vi "Prepend String Length.vi"(7 "String":string, 9 "byte order":T1(ring)=enum."native, host order") -> (8 "Length-prefixed string":string)   [LabVIEW 2020, in "epl-network.lvlib"]
uses:
  epl-network.lvlib
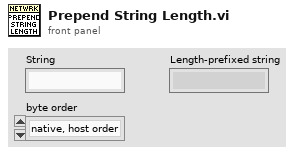
[diagram p1: front panel]
types:
  T1 = enum16{"big-endian, network order", "native, host order", "little-endian"}
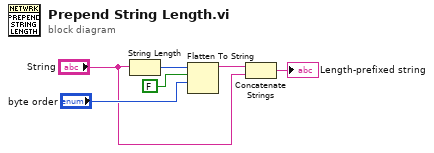
[diagram p0: block diagram]
diagram:
  n1 = String Length(string="String") -> (length=w2:i32)
  n2 = Flatten To String(anything=w2, prepend array or string size? (T)=FALSE, byte order (0:big-endian, network order)="byte order") -> (data string=w1:string)  [unwired: 1 in, 2 out]
  n3 = Concatenate Strings(w1, "String") -> (→"Length-prefixed string":string)
